vi "RectROIfromMatchPOS (SubVI).vi"(6 "ROI Rect Descriptor":T5={"Global Rectangle"=[0, 132, 2592, 1180], "Contours"=[{"ID"=enum."External", "Type"=12, "Coordinates"=[5, 132, 2612, 1180, 0]}]} {"Contours"."Type" items=["No Selection", "Point", "Line", "Rectangle", "Oval", "Polygon", "Freehand Region", "Annulus", "Unused2", "Unused3", "Broken Line", "Freehand Line", "Rotated Rectangle"]}, 9 "Calibrated Image":T1, 10 "Pattern Match Settings":T4={"Algorithm"=2, "Number of Matches Requested"=1, "Minimum Match Score"=800.0, "SubPixel Accuracy"=TRUE, "Rotation Angle Ranges"=[], "Show Search Area"=FALSE, "Show Result"=TRUE} {"Rotation Angle Ranges"."End" format="%.1f"; "Rotation Angle Ranges"."Start" format="%.1f"; "Minimum Match Score" min=0 max=1000 format="%.2f"; "Number of Matches Requested" min=1; "Algorithm" items=["All", "Low Discrepancy Sampling", "Grayscale Value Pyramid", "Gradients Pyramid"]}, 11 "Template in":T1) -> (1 "output Rect ROI":T2, 2 "Pattern Matches (pixel)":T3(array[cluster]) {"Bounding Box"."y" format="%.2f"; "Bounding Box"."x" format="%.2f"; "Position"."y" format="%.2f"; "Position"."x" format="%.2f"; "Score" format="%.2f"; "Scale" format="%.2f"; "Angle" format="%.2f"}, 3 "Calibated image out":T1)   [LabVIEW 2016]
uses:
  <vilib>/vision/Image Controls.llb/IMAQ Image.ctl
  <vilib>/vision/NI_Vision_Development_Module.lvlib
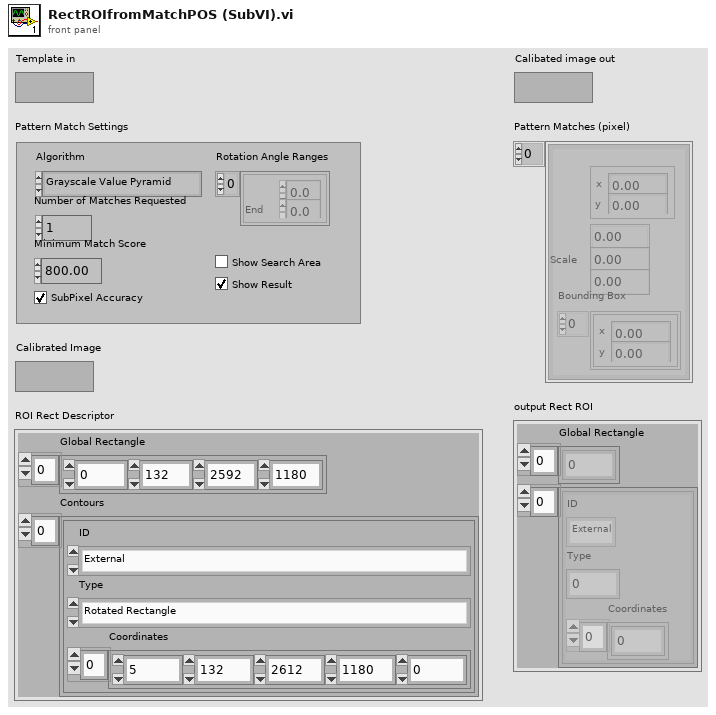
[diagram p1: front panel]
types:
  T1 = typedef "IMAQ Image.ctl" = refnum<image>
  T2 = cluster{"Global Rectangle":i32[], cluster{"ID":enum32{"External", "Internal"}, "Type":u32, "Coordinates":i32[]}[]}
  T3 = cluster{"Position":cluster{"x":sgl, "y":sgl}, "Angle":sgl, "Scale":sgl, "Score":sgl, "Bounding Box":cluster{"x":sgl, "y":sgl}[]}[]
  T4 = cluster{"Algorithm":i32, "Number of Matches Requested":i32, "Minimum Match Score":sgl, "SubPixel Accuracy":bool, "Rotation Angle Ranges":cluster{"Start":sgl, "End":sgl}[], "Show Search Area":bool, "Show Result":bool}
  T5 = cluster{"Global Rectangle":i32[], "Contours":cluster{"ID":enum32{"External", "Internal"}, "Type":u32, "Coordinates":i32[]}[]}
  T6 = cluster{"ID":enum32{"External", "Internal"}, "Type":u32, "Coordinates":i32[]}[]
  T7 = cluster{"ID":enum32{"External", "Internal"}, "Type":u32, "Coordinates":i32[]}
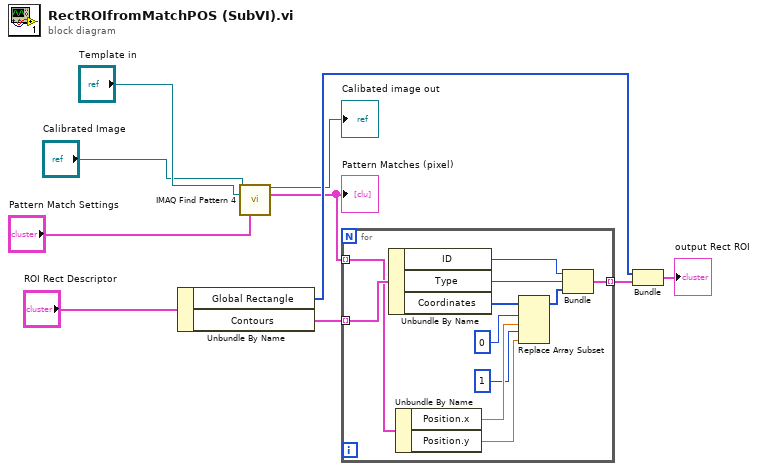
[diagram p0: block diagram]
diagram:
  n1 = Unbundle By Name("ROI Rect Descriptor") -> ("Global Rectangle"=w7:i32[], "Contours"=w8:T6)
  n2 = call "IMAQ Find Pattern 4"("Image"="Calibrated Image", "Template"="Template in", "Settings"="Pattern Match Settings") -> ("Image Out"=→"Calibated image out":T1, "Matches (pixel)"=w6:T3)  [unwired: 6 in, 5 out]
  "Pattern Matches (pixel)" <- w6
  n3 = for {
    tunnel: w6 -> [w15] mode=indexing
    tunnel: w8 -> [w21] mode=indexing
    tunnel: [w16] -> w9 mode=indexing
    n4 = Unbundle By Name(w21) -> ("ID"=w17:enum32{"External", "Internal"}, "Type"=w18:u32, "Coordinates"=w19:i32[])
    n5 = Unbundle By Name(w15) -> ("Position.x"=w14:sgl, "Position.y"=w13:sgl)
    n6 = Replace Array Subset(array=w19, new element #1=w14, index #1=0 ("index"), new element #2=w13, index #2=1 ("index")) -> (w20:i32[])
    n7 = Bundle("ID"=w17, "Type"=w18, "Coordinates"=w20) -> (w16:T7)  [unwired: 1 in]
  }
  n8 = Bundle("Global Rectangle"=w7, w9) -> (→"output Rect ROI":T2)  [unwired: 1 in]
